vi "OpenDevice.vi"(10 "pIdentifier":i64, 11 "error in (no error)":errorcluster) -> (1 "handle":i64, 2 "retrun type":i32, 3 "error out":errorcluster)   [LabVIEW 2016]
uses:
  MVSDKmd.dll
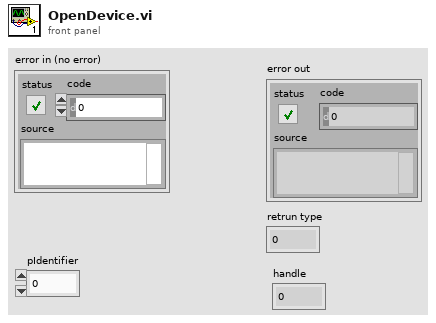
[diagram p1: front panel]
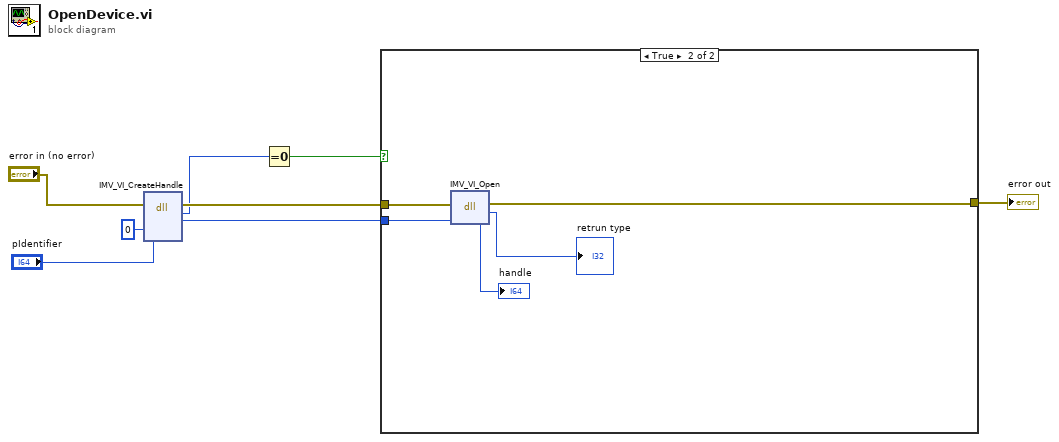
[diagram p0: block diagram]
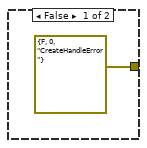
[diagram p2: hidden frame]
diagram:
  n1 = dll-call lib="MVSDKmd.dll" fn="IMV_VI_CreateHandle"(error in="error in (no error)", "mode"=0, "pIdentifier"="pIdentifier") -> (error out=w4:errorcluster, "return type"=w2:i32, "handle"=w6:i64)  [unwired: 5 in, 1 out]
  n2 = Equal To 0?(x=w2) -> (x = 0?=w1:bool)
  n3 = case shown="True" w1 {
    tunnel: w6 -> [_ w14]
    tunnel: w4 -> [_ w13]
    tunnel: [errorcluster {"status"=FALSE, "code"=0, "source"="CreateHandleError"} ("error out") w11] -> w3
    frame False {
    }
    frame True {
      n4 = dll-call lib="MVSDKmd.dll" fn="IMV_VI_Open"(error in=w13, "handle"=w14) -> (error out=w11:errorcluster, "return type"=→"retrun type":i32, "handle"=→"handle":i64)  [unwired: 2 in, 1 out]
    }
  }
  "error out" <- w3
